vi "niDTS BT INSTR RX Configure Payload.vi"(8 "error in (no error)":errorcluster, 11 "niDTS BT INSTR RX in":refnum<class "niDTS BT INSTR RX.lvclass">) -> (0 "error out":errorcluster, 3 "niDTS BT INSTR RX out":refnum<class "niDTS BT INSTR RX.lvclass">)   [LabVIEW 2015, in "niDTS BT.lvlib" / "niDTS BT INSTR RX.lvclass"]
uses:
  niDTS BT INSTR RX.lvclass
  niDTS BT INSTR RX.lvclass/niDTS BT INSTR RX.ctl
  RiviInstDriver/niRfsgBT/Objects/niRfsgBt.lvclass
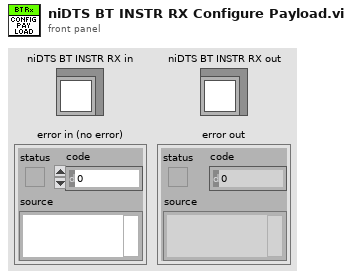
[diagram p1: front panel]
types:
  T1 = cluster{"LCh":i32, "HeaderFlowControlBit":bool, "Length":i32}
  T2 = typedef "niRfsgBT.lvclass/niRfsgBT INC Handle.ctl" = refnum<data-value>
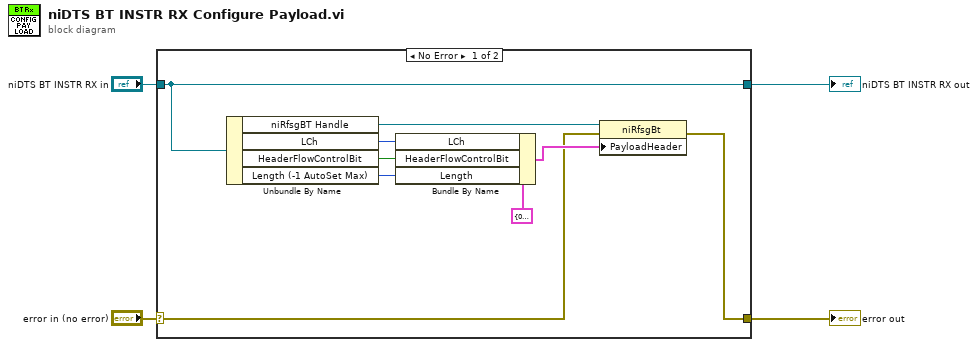
[diagram p0: block diagram]
diagram:
  n1 = case shown="No Error" "error in (no error)" {
    selector: "error in (no error)" -> [w6 w14]
    tunnel: [w5 w14] -> w3
    tunnel: [w13 w15] -> w1
    tunnel: "niDTS BT INSTR RX in" -> [w13 w15]
    frame No Error {
      n2 = Unbundle By Name(w13) -> ("niRfsgBT Handle"=w12:T2, "LCh"=w10:i32, "HeaderFlowControlBit"=w9:bool, "Length (-1 AutoSet Max)"=w8:i32)
      n3 = Bundle By Name(cluster=T1 {"LCh"=0, "HeaderFlowControlBit"=FALSE, "Length"=0} ("SOURce:RFSG:BLUetooth:PACKet:PAYLoad:HEADer_A"), "LCh"=w10, "HeaderFlowControlBit"=w9, "Length"=w8) -> (w7:T1)
      n4 = property class="niRfsgBt"(reference=w12, error in=w6, "PayloadHeader"=w7) -> (error out=w5:errorcluster)  [unwired: 1 out]
    }
    frame Error {
    }
  }
  "error out" <- w3
  "niDTS BT INSTR RX out" <- w1
